vi "Telnet Read Filter.vi"(4 "error in":errorcluster, 5 "unfiltered data in":string, 7 "Connection in":refnum<k5>) -> (0 "error out":errorcluster, 1 "Unfiltered data out":string, 2 "Data out":string, 3 "connection out":refnum<k5>)   [LabVIEW 2015]
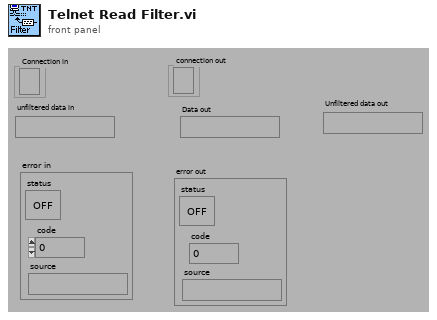
[diagram p1: front panel]
types:
  T1 = cluster{"command":enum16{"WILL", "WON'T", "DO", "DON'T"}, "option":u8}
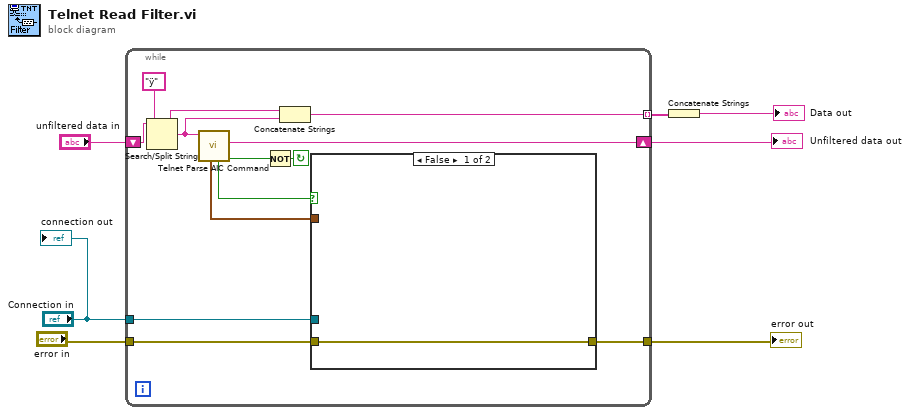
[diagram p0: block diagram]
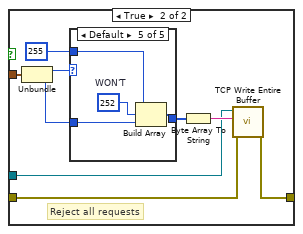
[diagram p2: hidden frame]
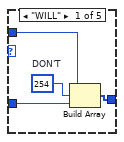
[diagram p3: hidden frame]
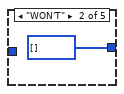
[diagram p4: hidden frame]
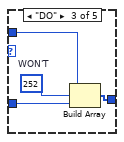
[diagram p5: hidden frame]
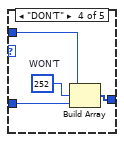
[diagram p6: hidden frame]
diagram:
  n1 = while {
    shift-right: [w13] -> w3
    shift-left: "unfiltered data in" -> [w19]
    tunnel: "error in" -> [w17]
    tunnel: "Connection in" -> [w15]
    tunnel: [w16] -> w5
    tunnel: [w14] -> w2 mode=indexing
    stop <- w18 continue-if-true
    n2 = Search/Split String(string=w19, search string/char (-)="ÿ" ("regular expression")) -> (substring before match=w9:string, match + rest of string=w8:string)  [unwired: 1 in, 1 out]
    n3 = call "Telnet Parse AIC Command.vi"("AIC sequence"=w8) -> ("error"=w12:bool, "after sequence"=w13:string, "option negotiation"=w11:bool, "option info"=w10:T1)  [unwired: 4 in, 3 out]
    n4 = Not(x=w12) -> (.not. x?=w18:bool)
    n5 = Concatenate Strings(w9, w8) -> (w14:string)
    n6 = case shown="False" w11 {
      tunnel: w10 -> [_ w30]
      tunnel: w17 -> [w21 w25]
      tunnel: [w21 w24] -> w16
      tunnel: w15 -> [_ w23]
      frame False {
      }
      frame True {
        # "Reject all requests"
        n7 = Unbundle(w30) -> ("command"=w29:enum16{"WILL", "WON'T", "DO", "DON'T"}, "option"=w28:u8)
        n8 = case shown="Default" w29 {
          tunnel: w28 -> [w34 _ w39 w43 w46]
          tunnel: [w32 u8[] [] w37 w41 w45] -> w27
          tunnel: u8 255 -> [w31 _ w36 w40 w44]
          frame "WILL" {
            w33 = u8 254  # DON'T
            n9 = Build Array(w31, w33, w34) -> (w32:u8[])
          }
          frame "WON'T" {
          }
          frame "DO" {
            w38 = u8 252  # WON'T
            n10 = Build Array(w36, w38, w39) -> (w37:u8[])
          }
          frame "DON'T" {
            w42 = u8 252  # WON'T
            n11 = Build Array(w40, w42, w43) -> (w41:u8[])
          }
          frame Default {
            w47 = u8 252  # WON'T
            n12 = Build Array(w44, w47, w46) -> (w45:u8[])
          }
        }
        n13 = Byte Array To String(unsigned byte array=w27) -> (string=w26:string)
        n14 = call "TCP Write Entire Buffer.vi"("error in (no error)"=w25, "data in"=w26, "connection ID"=w23) -> ("error out"=w24:errorcluster)  [unwired: 6 in, 2 out]
      }
    }
  }
  "Unfiltered data out" <- w3
  "error out" <- w5
  n15 = Concatenate Strings(w2) -> (→"Data out":string)
  "connection out" <- "Connection in"
